vi "Update State Name 2.vi"(8 "error in (no error)":errorcluster, 10 "State":string, 11 "Channel Ref in":T1 format="%.0x") -> (0 "error out":errorcluster, 3 "Channel Ref out":T1=18446744073709551615 format="%.0x")   [LabVIEW 2017, in "Switch Scripting.lvlib"]
uses:
  Switch Scripting.lvlib
  NationalInstruments.VeriStand.SystemDefinitionAPI
  Shared/Constants.vi
  Shared/Switch Shared.lvlib
  <vilib>/NI Veristand/Custom Device API/Custom Device Item Ref.ctl
  <vilib>/NI VeriStand/Custom Device API/Custom Device API.lvlib
panel:
  in  "New State Name":string
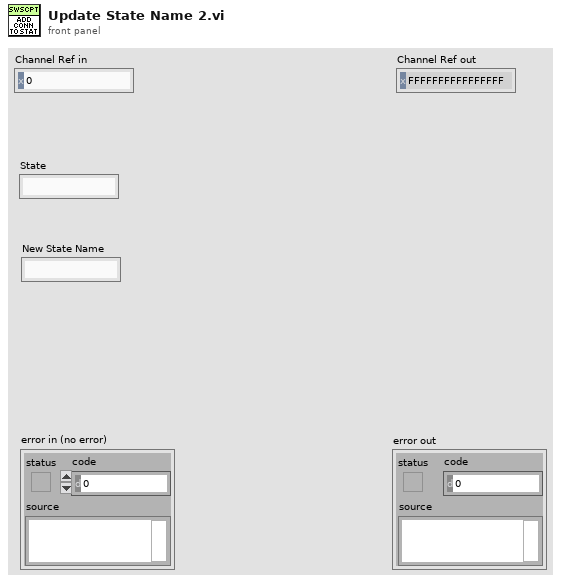
[diagram p1: front panel]
types:
  T1 = typedef "Custom Device API.lvlib/Custom Device Item Ref.ctl" = u64
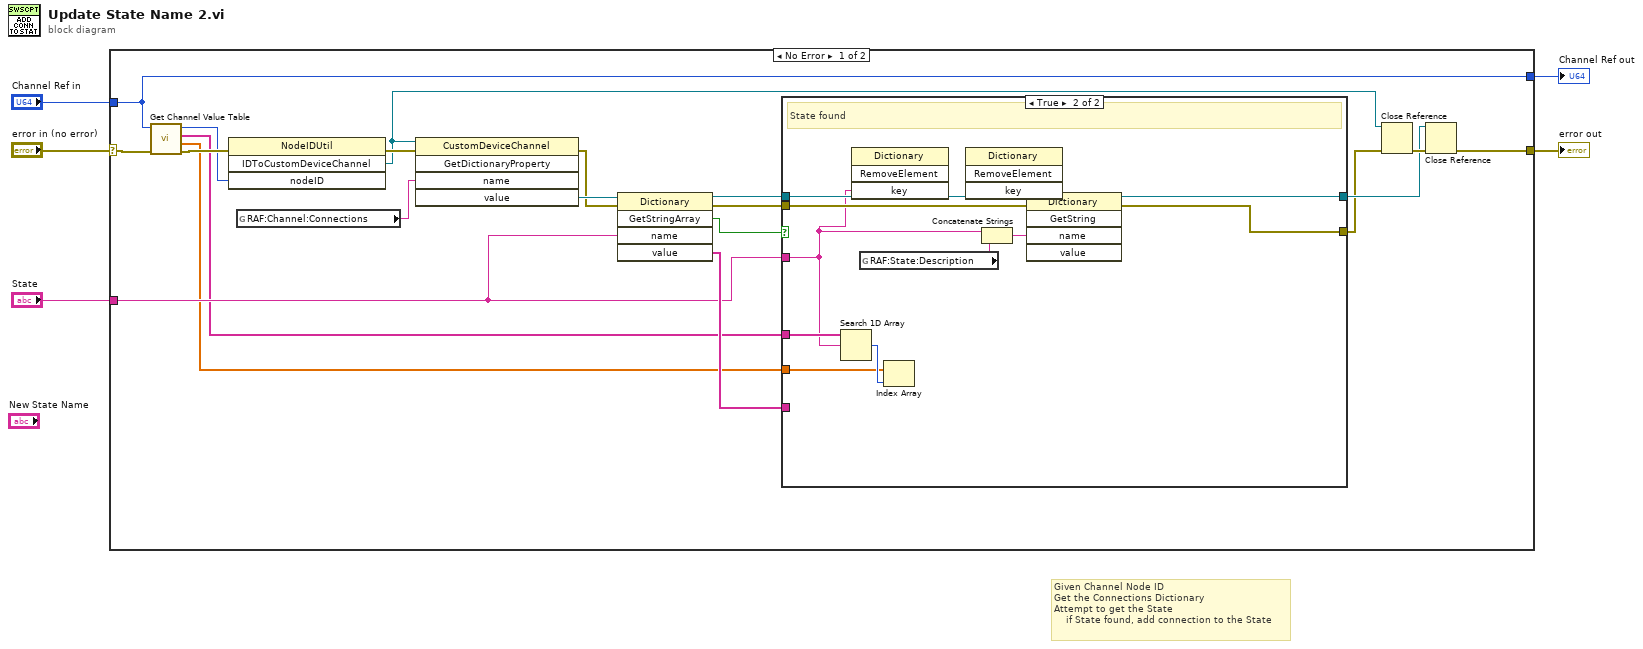
[diagram p0: block diagram]
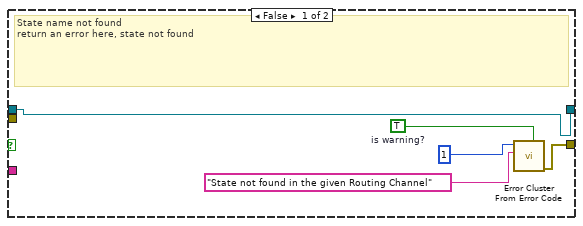
[diagram p2: hidden frame]
diagram:
  # "Given Channel Node ID\nGet the Connections Dictionary\nAttempt to get the State\n    if State found, add connection to the State"
  n1 = case shown="No Error" "error in (no error)" {
    selector: "error in (no error)" -> [w11 w42]
    tunnel: [w25 w42] -> w4
    tunnel: "Channel Ref in" -> [w9 w41]
    tunnel: [w9 w41] -> w2
    tunnel: "State" -> [w12 _]
    frame No Error {
      n2 = call "Get Channel Value Table.vi"("error in (no error)"=w11, "Channel Ref in"=w9) -> ("error out"=w10:errorcluster, "Values"=w6:dbl[], "States"=w7:string[], "Channel Ref out"=w8:T1)  [unwired: 6 in]
      n3 = invoke class="NodeIDUtil" method="IDToCustomDeviceChannel"(error in=w10, "nodeID"=w8) -> (error out=w23:errorcluster, "IDToCustomDeviceChannel"=w13:refnum<k24>)  [unwired: 2 in, 2 out]
      n4 = global read "Constants.vi" "RAF:Channel:Connections"() -> (w14:string)
      n5 = invoke class="CustomDeviceChannel" method="GetDictionaryProperty"(reference=w13, error in=w23, "name"=w14) -> (error out=w20:errorcluster, "value"=w21:refnum<k24>)  [unwired: 2 in, 3 out]
      n6 = invoke class="Dictionary" method="GetStringArray"(reference=w21, error in=w20, "name"=w12) -> (reference out=w17:refnum<k24>, error out=w18:errorcluster, "GetStringArray"=w19:bool, "value"=w22:string[])  [unwired: 2 in, 1 out]
      n7 = case shown="True" w19 {
        tunnel: w22 -> [_ _]
        tunnel: w18 -> [_ w33]
        tunnel: [w27 w34] -> w15
        tunnel: w17 -> [w26 w38]
        tunnel: [w26 w35] -> w16
        tunnel: w12 -> [_ w32]
        tunnel: w7 -> [_ w37]
        tunnel: w6 -> [_ w36]
        frame False {
          w29 = TRUE  # is warning?
          # "State name not found\nreturn an error here, state not found"
          n8 = call <vilib>:"Error Cluster From Error Code.vi"("is warning? (False)"=w29, "error message (\"\")"="State not found in the given Routing Channel" ("error message (\"\")"), "error code (0)"=1) -> ("error out"=w27:errorcluster)  [unwired: 6 in]
        }
        frame True {
          # "State found"
          n9 = Search 1D Array(1D array=w37, element=w32) -> (index of element=w40:i32)  [unwired: 1 in]
          n10 = invoke class="Dictionary" method="RemoveElement"("key"=w32) -> ()  [unwired: 3 in, 4 out]
          n11 = global read "Constants.vi" "RAF:State:Description"() -> (w39:string)
          n12 = Index Array(array=w36, index=w40) -> ()  [unwired: 1 out]
          n13 = invoke class="Dictionary" method="RemoveElement"() -> ()  [unwired: 4 in, 4 out]
          n14 = Concatenate Strings(w32, w39) -> (w31:string)
          n15 = invoke class="Dictionary" method="GetString"(reference=w38, error in=w33, "name"=w31) -> (reference out=w35:refnum<k24>, error out=w34:errorcluster)  [unwired: 2 in, 3 out]
        }
      }
      n16 = Close Reference(reference=w13, error in (no error)=w15) -> (error out=w24:errorcluster)
      n17 = Close Reference(reference=w16, error in (no error)=w24) -> (error out=w25:errorcluster)
    }
    frame Error {
    }
  }
  "Channel Ref out" <- w2
  "error out" <- w4
